vi "TTA_MATLAB_Generic_Test_Function_Call.vi"(0 "Tile Section":enum16{"RFIC", "Tx", "Rx"}(ring), 1 "Instrument Cluster In":T1, 5 "Sub-Function Name":string, 7 "Complete Settings Cluster":T2, 11 "error in":errorcluster) -> (4 "SubTestSuccess":dbl[](array[numeric]), 6 "SubTestSuccess":bool[](array[boolean]), 12 "Instrument Cluster Out":T1, 15 "error out":errorcluster)   [LabVIEW 2016]
uses:
  TTA_Controls/TTA_Control_Complete_Settings_Cluster.ctl
  TTA_Controls/TTA_Control_Instrument_Cluster.ctl
  TTA_Globals/TTA_Global_Complete_Settings.vi
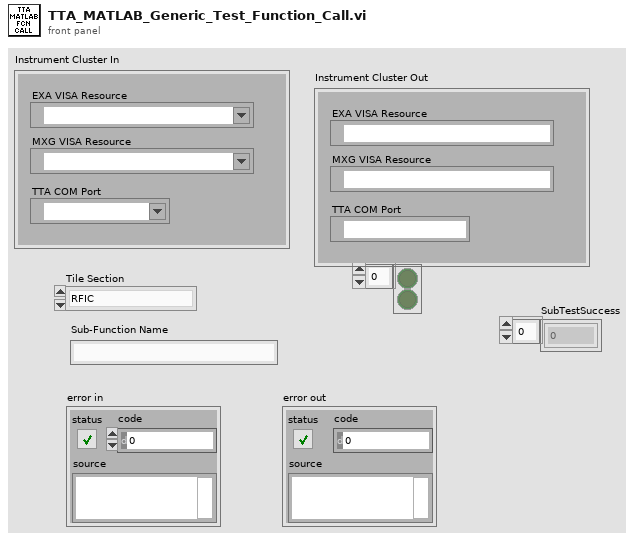
[diagram p1: front panel]
types:
  T1 = typedef "TTA_Control_Instrument_Cluster.ctl" = cluster{"EXA VISA Resource":refnum<visa-resource-name>, "MXG VISA Resource":refnum<visa-resource-name>, "TTA COM Port":refnum<visa-resource-name>}
  T2 = typedef "TTA_Control_Complete_Settings_Cluster.ctl" = cluster{"Brief Cluster":cluster{"STM Firmware File":string, "STM Firmware Address":string, "Required SW Version":string, "Template Used":string}, "Instrument Setting Cluster":cluster{"BDSFreq":dbl, "BDS Amp":dbl, "TxRFCal_Freq":dbl, "TxRFCal_Amp":dbl, "RxRFCal_Freq":dbl, "RxRFCal_Freq":dbl, "TxIF_Freq":dbl, "TxIF_Amp":dbl, "Tx_Output_Power_Signal_Freq":dbl, "Tx_ACPR_Signal_Freq":dbl, "Rx_RF_Freq":dbl, "Rx_RF_Amp":dbl, "Rx_Output_Power_Signal_Freq":dbl, "Rx_Output_Power_Sense_Freq":dbl}, "PAL Calibration\nInputs Cluster":cluster{"Amplitude Range\nMax(dBm)":dbl, "Amplitude Range\nMin(dBm)":dbl, "Amplitude Least\nCriteria (dBm)":dbl, "Frequency 1":dbl, "Frequency 2":dbl, "Frequency 3":dbl, "CAL Amplitude\nDecrement (dB)":dbl, "CAL Amplitude\nIncrement(dB)":dbl, "DownloadFile":string}, "TxOffset Cal Cluster":cluster{"Tx1 Offset (dB)":dbl, "Tx2 Offset (dB)":dbl, "Tx3 Offset (dB)":dbl, "Tx4 Offset (dB)":dbl, "Total RF Tx Loss (dB)":dbl}, "RxOffset Cal Cluster":cluster{"Rx1 Offset (dB)":dbl, "Rx2 Offset (dB)":dbl, "Rx3 Offset (dB)":dbl, "Rx4 Offset (dB)":dbl, "Total RF Rx Loss (dB)":dbl}, "TX Output Power Settings Cluster":cluster{"Frequency Sweep (MHz)":dbl[], "Sig Gen \nPower (dBm)":dbl, "Span (kHz)":dbl, "RBW (Hz)":dbl, "Ref Level (dBm)":dbl, "Low Power \nLimit":dbl, "High Power \nLimit":dbl, "DigAtt Max":dbl, "DigAtt Min":dbl}, "Tx ACPR Settings Cluster":cluster{"ACPR Filename":string, "Sampling Rate":dbl, "Power (dBm)":dbl, "IF Frequency Sweep (MHz)":dbl[], "State Name":string, "Mechanical\nAttenuation":dbl, "RefLevel Offset":dbl, "Amplitude Range\nMax (dBm)":dbl, "Amplitude Range\nMin (dBm)":dbl, "Cal Amp \nIncrement (dB)":dbl, "Cal Amp\nDecrement (dB)":dbl}, "Power Cal Cluster":cluster{"Power List (dBm)":dbl[], "Frequency (MHz)":dbl[], "Cal Decrement (dB)":dbl, "Cal Increment (dB)":dbl}, "Rx Received Power Settings Cluster":cluster{"Frequency Sweep (MHz)":dbl[], "Power (dBm)":dbl, "Span (kHz)":dbl, "RBW (Hz)":dbl, "Ref Level":dbl, "Low Power \nLimit (dBm)":dbl, "High Power\nLimit (dBm)":dbl}, "Tx Output Power Criteria Cluster":cluster{"CH1-TX1 \nMin":dbl, "CH1-TX1\nMax":dbl, "CH1-TXx3\nMin ":dbl, "CH1-TXx3\nMax":dbl, "CH2-TX1\nMin":dbl, "CH2-TX1\nMax":dbl, "CH2-TXx3\nMin":dbl, "CH2-TXx3\nMax":dbl}, "Tx ACPR Criteria Cluster":cluster{"Min Inband":dbl, "Max Close Outband":dbl, "Max Far Outband":dbl}, "Rx Output Power Criteria Cluster":cluster{"CH1-RX1 \nMin":dbl, "CH1-RX1 \nMax":dbl, "CH1-RXx3 \nMin":dbl, "CH1-RXx3\nMax":dbl, "CH2-RX1\nMin":dbl, "CH2-RX1\nMax":dbl, "CH2-RXx3\nMin":dbl, "CH2-RXx3\nMax":dbl}}
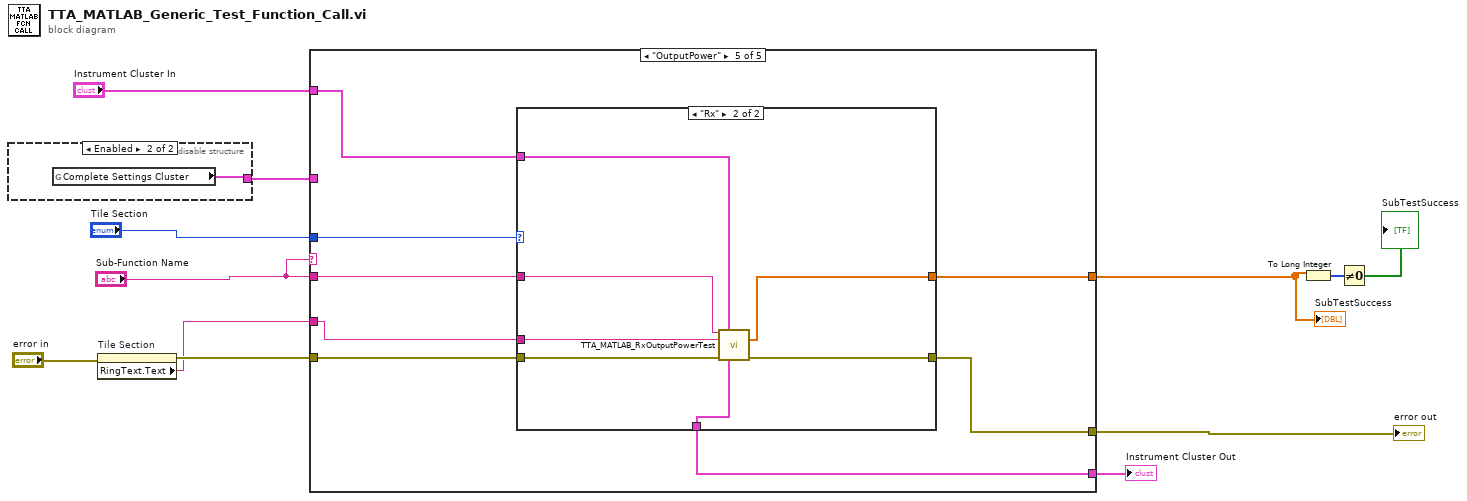
[diagram p0: block diagram]
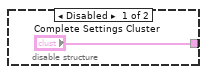
[diagram p2: hidden frame]
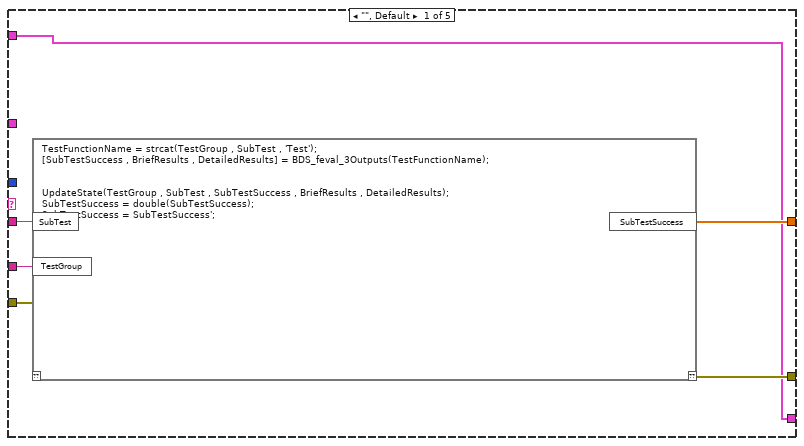
[diagram p3: hidden frame]
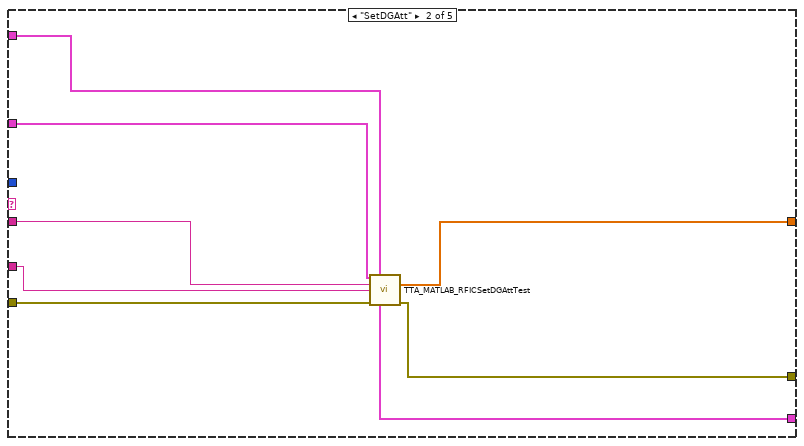
[diagram p4: hidden frame]
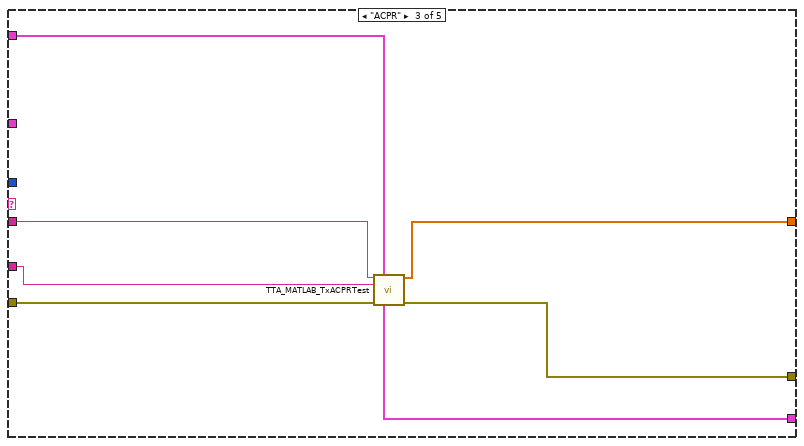
[diagram p5: hidden frame]
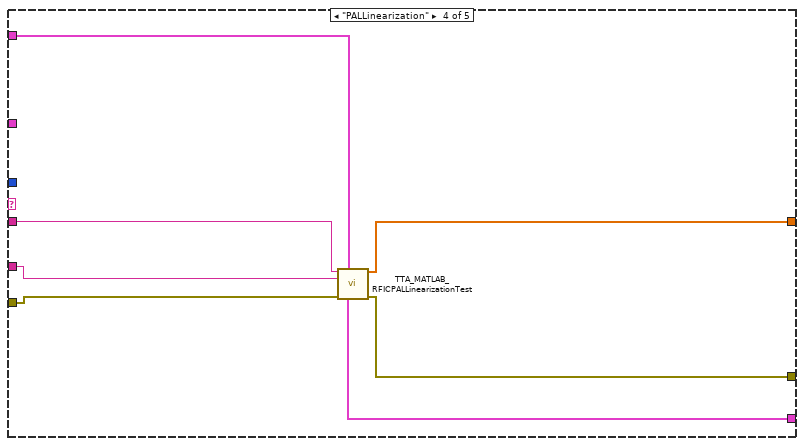
[diagram p6: hidden frame]
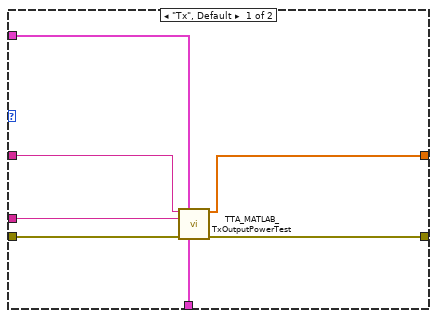
[diagram p7: hidden frame]
diagram:
  n1 = disable-structure shown="Enabled" {
    disable-tunnel: ["Complete Settings Cluster" w14] -> w4
    frame Disabled {
    }
    frame Enabled {
      n2 = global read "TTA_Global_Complete_Settings.vi" "Complete Settings Cluster"() -> (w14:T2)
    }
  }
  n3 = property on="Tile Section" class="Enum (strict)"(error in="error in") -> (error out=w10:errorcluster, "RingText.Text"=w9:string)  [unwired: 1 in, 1 out]
  n4 = case shown="\"OutputPower\"" "Sub-Function Name" {
    tunnel: "Sub-Function Name" -> [w20 w22 w32 w38 w48]
    tunnel: [w19 w26 w30 w39 w44] -> w12
    tunnel: w10 -> [w18 w27 w35 w40 w49]
    tunnel: w9 -> [w17 w21 w31 w37 w47]
    tunnel: [w16 w23 w29 w36 w43] -> w6
    tunnel: w4 -> [_ w28 _ _ _]
    tunnel: "Instrument Cluster In" -> [w15 w25 w34 w42 w46]
    tunnel: [w15 w24 w33 w41 w45] -> w2
    tunnel: "Tile Section" -> [_ _ _ _ w50]
    frame "", Default {
      n5 = script code="TestFunctionName = strcat(TestGroup , SubTest , 'Test');\n[SubTestSuccess , BriefResults , DetailedResults] = BDS_feval_3Outputs(TestFunctionName);\n\n\nUpdateState(TestGroup , SubTest , SubTestSuccess , BriefResults , DetailedResults);\nSubTestSuccess = double(SubTestSuccess);\nSubTestSuccess = SubTestSuccess';"("??"=w18, "SubTest"=w20, "TestGroup"=w17) -> ("??"=w19:errorcluster, "SubTestSuccess"=w16:dbl[])
    }
    frame "SetDGAtt" {
      n6 = call "TTA_MATLAB_RFICSetDGAttTest.vi"("Complete Settings Cluster"=w28, "Instrument Cluster In"=w25, "Sub-Function Name"=w22, "Test Group"=w21, "error in"=w27) -> ("SubTestSuccess"=w23:dbl[], "Instrument Cluster Out"=w24:T1, "error out"=w26:errorcluster)  [unwired: 8 in]
    }
    frame "ACPR" {
      n7 = call "TTA_MATLAB_TxACPRTest.vi"("Sub-Function Name"=w32, "Instrument Cluster In"=w34, "Test Group"=w31, "error in"=w35) -> ("SubTestSuccess"=w29:dbl[], "Instrument Cluster Out"=w33:T1, "error out"=w30:errorcluster)  [unwired: 9 in]
    }
    frame "PALLinearization" {
      n8 = call "TTA_MATLAB_RFICPALLinearizationTest.vi"("Sub-Function Name"=w38, "Instrument Cluster In"=w42, "Test Group"=w37, "error in"=w40) -> ("SubTestSuccess"=w36:dbl[], "Instrument Cluster Out"=w41:T1, "error out"=w39:errorcluster)  [unwired: 9 in]
    }
    frame "OutputPower" {
      n9 = case shown="\"Rx\"" w50 {
        tunnel: w49 -> [w57 w64]
        tunnel: w48 -> [w56 w63]
        tunnel: w47 -> [w55 w62]
        tunnel: w46 -> [w54 w61]
        tunnel: [w53 w60] -> w45
        tunnel: [w52 w58] -> w44
        tunnel: [w51 w59] -> w43
        frame "Tx", Default {
          n10 = call "TTA_MATLAB_TxOutputPowerTest.vi"("Sub-Function Name"=w56, "Instrument Cluster In"=w54, "Test Group"=w55, "error in"=w57) -> ("SubTestSuccess"=w51:dbl[], "Instrument Cluster Out"=w53:T1, "error out"=w52:errorcluster)  [unwired: 9 in]
        }
        frame "Rx" {
          n11 = call "TTA_MATLAB_RxOutputPowerTest.vi"("Sub-Function Name"=w63, "Instrument Cluster In"=w61, "Test Group"=w62, "error in"=w64) -> ("SubTestSuccess"=w59:dbl[], "Instrument Cluster Out"=w60:T1, "error out"=w58:errorcluster)  [unwired: 8 in, 1 out]
        }
      }
    }
  }
  "error out" <- w12
  "SubTestSuccess" <- w6
  "Instrument Cluster Out" <- w2
  n12 = To Long Integer(number=w6) -> (32bit integer=w8:i32[])
  n13 = Not Equal To 0?(x=w8) -> (x != 0?=→"SubTestSuccess":bool[])
